vi "variables.vi"() -> ()   [LabVIEW 2020]
panel:
  out "Numeric":i32
  in  "stop":bool
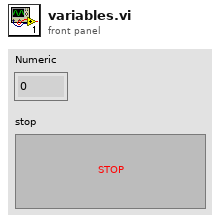
[diagram p1: front panel]
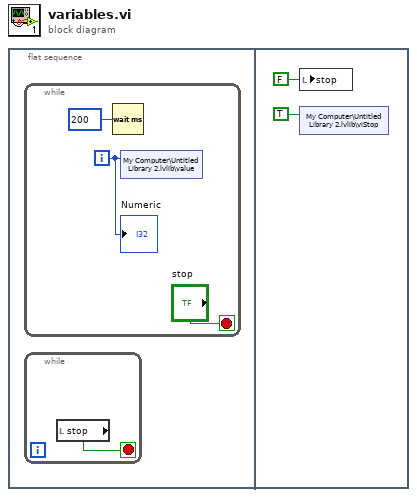
[diagram p0: block diagram]
diagram:
  n1 = flat-sequence {
    frame #0 {
      n2 = while {
        i -> [w3]
        stop <- "stop" stop-if-true
        n3 = Wait (ms)(milliseconds to wait=u32 200) -> ()  [unwired: 1 out]
        n4 = shared-variable "My Computer\\Untitled Library 2.lvlib\\value"(w3) -> ()  [unwired: 1 in, 1 out]
        "Numeric" <- w3
      }
      n5 = while {
        stop <- w1 stop-if-true
        n6 = local read "stop"() -> (w1:bool)
      }
    }
    frame #1 {
      n7 = local write "stop"(FALSE) -> ()
      n8 = shared-variable "My Computer\\Untitled Library 2.lvlib\\viStop"(TRUE ("viStop")) -> ()  [unwired: 1 in, 1 out]
    }
  }
